vi "Set Pixel Mode.vi"(8 "error in (no error)":errorcluster, 10 "colormode":i32, 11 "bitdepth":i32) -> (0 "error out":errorcluster, 3 "function return":u32)   [LabVIEW 2014, in "atmcd32d.lvlib"]
doc: "unsigned int WINAPI SetPixelMode(int bitdepth, int colormode);"
uses:
  atmcd32d.lvlib
  atmcd32d.dll
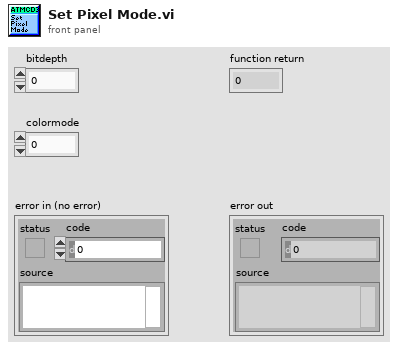
[diagram p1: front panel]
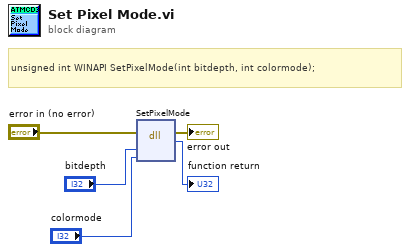
[diagram p0: block diagram]
diagram:
  # "unsigned int WINAPI SetPixelMode(int bitdepth, int colormode);"
  n1 = dll-call lib="C:/Users/Bakir/Documents/Lambda2-Testing/lib/Andorlib/atmcd32d.*" fn="SetPixelMode"(error in="error in (no error)", "bitdepth"="bitdepth", "colormode"="colormode") -> (error out=→"error out":errorcluster, →"function return":u32)  [unwired: 4 in, 1 out]
